vi "FiberWLC_CalcGiLi.vi"(10 "Lw1, Lw2, NRL (bp)":dbl[](array[numeric]), 11 "G1, G2, G3 (kT)":dbl[](array[numeric])) -> (2 "Li (bp)":dbl[](array[numeric]), 3 "Gi (kT)":dbl[](array[numeric]))   [LabVIEW 2018]
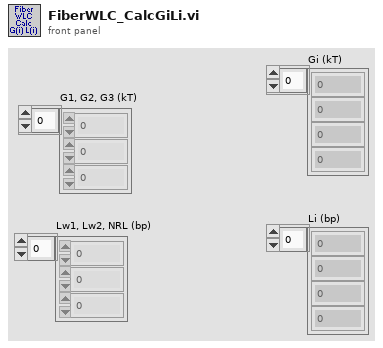
[diagram p1: front panel]
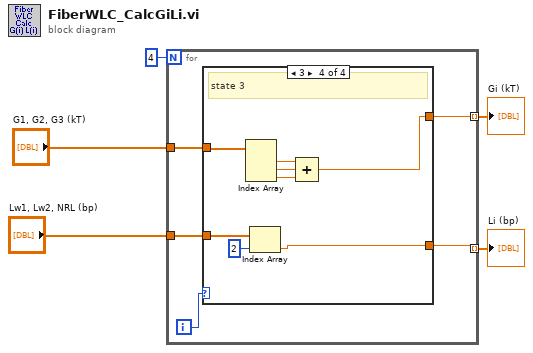
[diagram p0: block diagram]
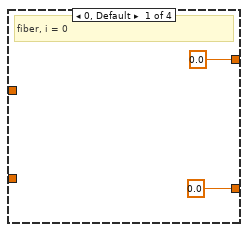
[diagram p2: hidden frame]
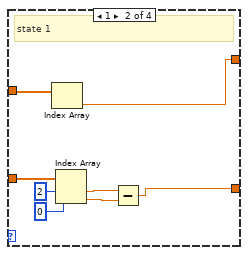
[diagram p3: hidden frame]
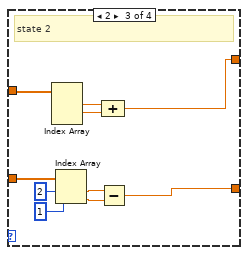
[diagram p4: hidden frame]
diagram:
  n1 = for {
    N: 4 -> [_]
    tunnel: "G1, G2, G3 (kT)" -> [w7]
    tunnel: "Lw1, Lw2, NRL (bp)" -> [w6]
    tunnel: [w9] -> w2 mode=indexing
    tunnel: [w8] -> w1 mode=indexing
    i -> [w10]
    n2 = case shown="3" w10 {
      tunnel: [0.0 w19 w26 w34] -> w9
      tunnel: [0.0 w14 w23 w35] -> w8
      tunnel: w7 -> [_ w20 w30 w38]
      tunnel: w6 -> [_ w18 w28 w36]
      frame 0, Default {
        # "fiber, i = 0"
      }
      frame 1 {
        # "state 1"
        n3 = Index Array(array=w20) -> (element=w19:dbl)  [unwired: 1 in]
        n4 = Index Array(array=w18, index #1=2 ("index"), index #2=0 ("index")) -> (element #1=w16:dbl, element #2=w15:dbl)
        n5 = Subtract(x=w16, y=w15) -> (x-y=w14:dbl)
      }
      frame 2 {
        # "state 2"
        n6 = Index Array(array=w30) -> (element #1=w29:dbl, element #2=w25:dbl)  [unwired: 3 in, 1 out]
        n7 = Index Array(array=w28, index #1=2 ("index"), index #2=1 ("index")) -> (element #1=w27:dbl, element #2=w22:dbl)
        n8 = Subtract(x=w27, y=w22) -> (x-y=w23:dbl)
        n9 = Compound Arithmetic op=ADD(w29, w25) -> (w26:dbl)
      }
      frame 3 {
        # "state 3"
        n10 = Index Array(array=w38) -> (element #1=w37:dbl, element #2=w33:dbl, element #3=w31:dbl)  [unwired: 3 in]
        n11 = Index Array(array=w36, index=2) -> (element=w35:dbl)
        n12 = Compound Arithmetic op=ADD(w37, w33, w31) -> (w34:dbl)
      }
    }
  }
  "Gi (kT)" <- w2
  "Li (bp)" <- w1
